vi "Check File Existence.vi"(8 "error in (no error)":errorcluster, 11 "File Parser Interface in":refnum<class "File Parser Interface.lvclass">) -> (0 "error out":errorcluster, 3 "File Parser Interface out":refnum<class "File Parser Interface.lvclass">)   [LabVIEW 2018, in "File Parser Interface.lvlib" / "File Parser Interface.lvclass"]
uses:
  File Parser Interface.lvclass
  File Parser Interface.lvclass/File Parser Interface.ctl
  Read File Path.vi
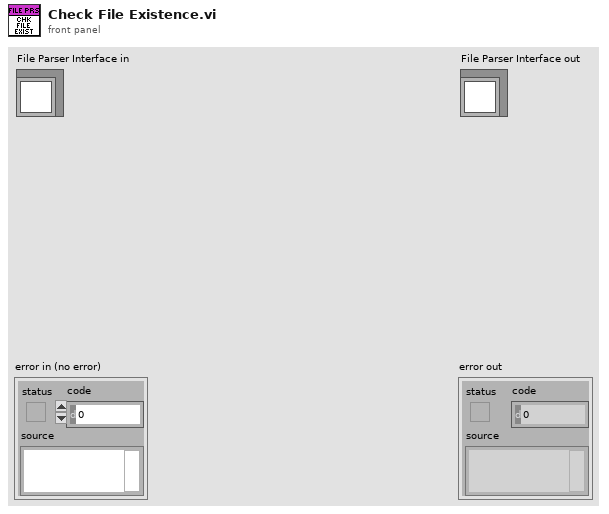
[diagram p1: front panel]
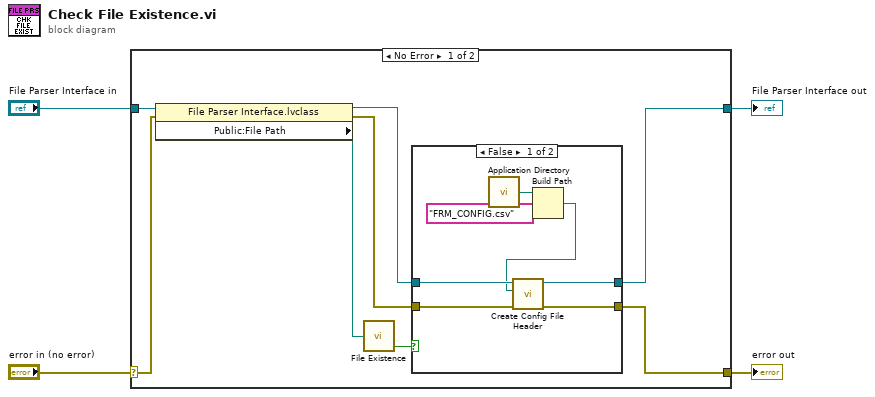
[diagram p0: block diagram]
diagram:
  n1 = case shown="No Error" "error in (no error)" {
    selector: "error in (no error)" -> [w11 w23]
    tunnel: [w5 w23] -> w3
    tunnel: [w6 w22] -> w1
    tunnel: "File Parser Interface in" -> [w12 w22]
    frame No Error {
      n2 = property class="File Parser Interface.lvclass"(reference=w12, error in=w11) -> (reference out=w8:refnum<class "File Parser Interface.lvclass">, error out=w9:errorcluster, "Public:File Path"=w7:path)
      n3 = call "File Existence.vi"("Path"=w7) -> ("exists"=w10:bool)  [unwired: 1 out]
      n4 = case shown="False" w10 {
        tunnel: w9 -> [w19 w20]
        tunnel: w8 -> [w18 w21]
        tunnel: [w17 w21] -> w6
        tunnel: [w16 w20] -> w5
        frame False {
          n5 = call <vilib>:"Application Directory.vi"() -> ("Application Directory"=w15:path)
          n6 = Build Path(base path=w15, name or relative path="FRM_CONFIG.csv") -> (appended path=w13:path)
          n7 = call-dynamic "Create Config File Header.vi"("error in (no error)"=w19, "Path"=w13, "File Parser Interface in"=w18) -> ("error out"=w16:errorcluster, "File Parser Interface out"=w17:refnum<class "File Parser Interface.lvclass">)  [unwired: 7 in]
        }
        frame True {
        }
      }
    }
    frame Error {
    }
  }
  "error out" <- w3
  "File Parser Interface out" <- w1
